vi "Type conversion.vi"() -> ()   [LabVIEW 2014]
panel:
  out "Y":dbl[](array[numeric])
  out "size(s)":i32
  out "string":string
  out "unsigned byte array":u8[](array[numeric])
  out "Boolean array":bool[](array[boolean])
  out "number":u32
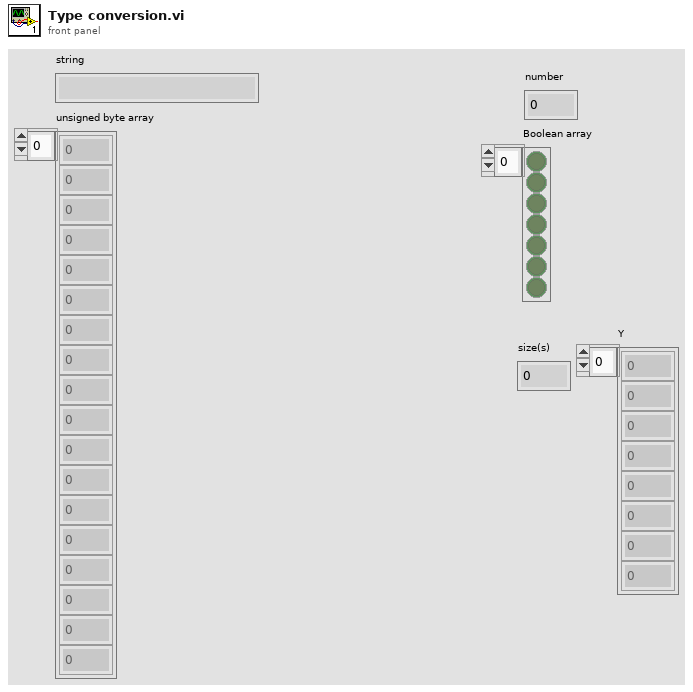
[diagram p1: front panel]
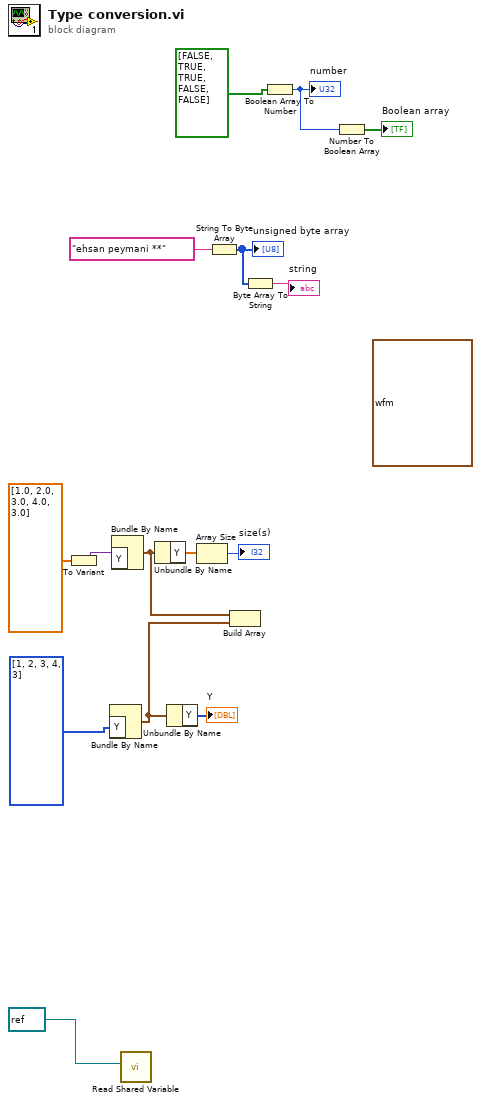
[diagram p0: block diagram]
diagram:
  (unwired) waveform(i32) {"t0"=timestamp(0 s since 1904-01-01), "dt"=1.0, "Y"=[]} ("Waveform")
  n1 = To Variant(anything=dbl[] [1.0, 2.0, 3.0, 4.0, 3.0]) -> (Variant=w2:variant)
  n2 = Bundle By Name("Y"=i32[] [1, 2, 3, 4, 3]) -> (w4:waveform(i32))  [unwired: 1 in]
  n3 = Bundle By Name("Y"=w2) -> (w5:waveform(dbl))  [unwired: 1 in]
  n4 = call "Read Shared Variable.vi"("Refnum"=refnum<k21> refnum) -> ()  [unwired: 8 in, 3 out]
  n5 = Unbundle By Name(w5) -> ("Y"=w9:dbl[])
  n6 = Unbundle By Name(w4) -> ("Y"=→"Y":i32[])
  n7 = Array Size(array=w9) -> (size(s)=→"size(s)":i32)
  n8 = String To Byte Array(string="ehsan peymani **") -> (unsigned byte array=w12:u8[])
  "unsigned byte array" <- w12
  n9 = Build Array(w5, w4) -> ()  [unwired: 1 out]
  n10 = Byte Array To String(unsigned byte array=w12) -> (string=→"string":string)
  n11 = Boolean Array To Number(Boolean array=bool[] [FALSE, TRUE, TRUE, FALSE, FALSE]) -> (number=w14:u32)
  "number" <- w14
  n12 = Number To Boolean Array(number=w14) -> (Boolean array=→"Boolean array":bool[])
